vi "UI Commands.vi"(8 "error in (no error)":errorcluster) -> (0 "error out":errorcluster, 2 "data":variant, 3 "Message":string)   [LabVIEW 2022 SP3]
uses:
  RT Global.vi
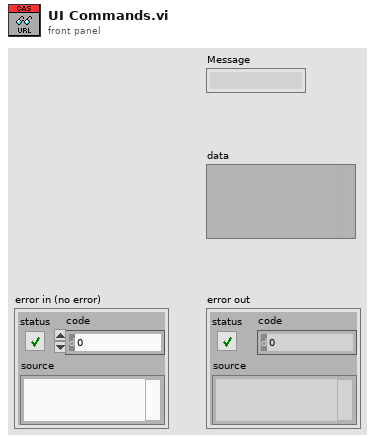
[diagram p1: front panel]
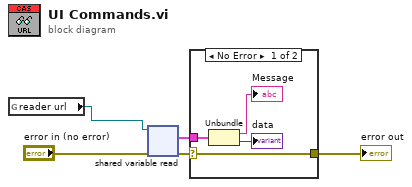
[diagram p0: block diagram]
diagram:
  n1 = global read "RT Global.vi" "reader url"() -> (w3:refnum<k21>)
  n2 = shared-variable-read(w3, "error in (no error)") -> (w2:errorcluster, w1:cluster{"Message":string, "Data":variant})  [unwired: 1 in, 2 out]
  n3 = case shown="No Error" w2 {
    selector: w2 -> [w9 w10]
    tunnel: [w9 w10] -> w4
    tunnel: w1 -> [w8 _]
    frame No Error {
      n4 = Unbundle(w8) -> ("Message"=→"Message":string, "Data"=→"data":variant)
    }
    frame Error {
    }
  }
  "error out" <- w4
